vi "Write cfg file folder.vi"(8 "error in (no error)":errorcluster, 10 "cfg file folder":path, 11 "[V] Sys Cfg Main in":refnum<class "[V] Sys Cfg Main.lvclass">) -> (0 "error out":errorcluster, 3 "[V] Sys Cfg Main out":refnum<class "[V] Sys Cfg Main.lvclass">)   [LabVIEW 2020, in "[V] Sys Cfg Main.lvlib" / "[V] Sys Cfg Main.lvclass"]
uses:
  [V] Sys Cfg Main.lvclass
  [V] Sys Cfg Main.lvclass/[V] Sys Cfg Main.ctl
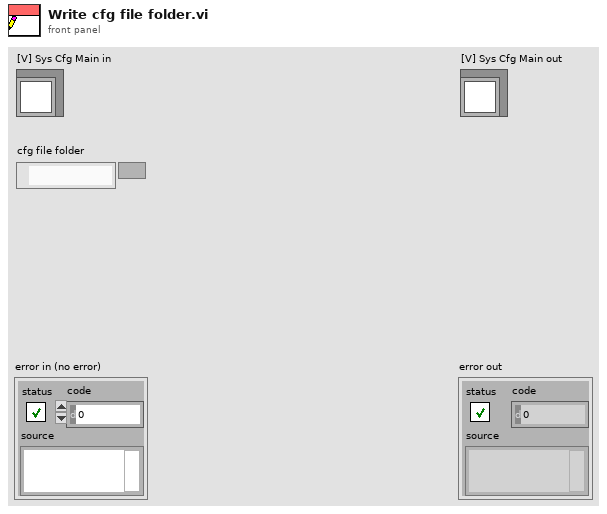
[diagram p1: front panel]
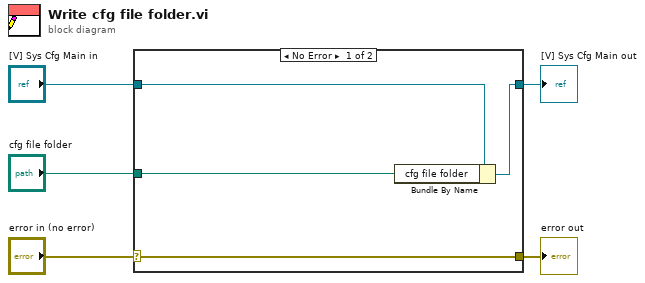
[diagram p0: block diagram]
diagram:
  n1 = case shown="No Error" "error in (no error)" {
    selector: "error in (no error)" -> [w9 w10]
    tunnel: [w9 w10] -> w4
    tunnel: [w7 w11] -> w2
    tunnel: "[V] Sys Cfg Main in" -> [w8 w11]
    tunnel: "cfg file folder" -> [w6 _]
    frame No Error {
      n2 = Bundle By Name(cluster=w8, "cfg file folder"=w6) -> (w7:refnum<class "[V] Sys Cfg Main.lvclass">)
    }
    frame Error {
    }
  }
  "error out" <- w4
  "[V] Sys Cfg Main out" <- w2
